vi "VIPM_Get Spec File Paths.vi"() -> (2 "Success?":bool, 3 "Spec Paths":path[](array[path]))   [LabVIEW 2019, in "Project.Dependencies Finder.lvlib" / "Dependency Source_VIPM.lvclass"]
doc: "Returns the paths to all Spec files in the JKI\\VIPM\\Cache folder."
uses:
  Dependency Source_VIPM.lvclass
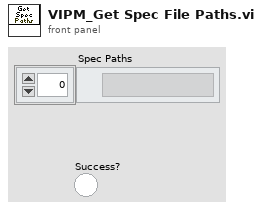
[diagram p1: front panel]
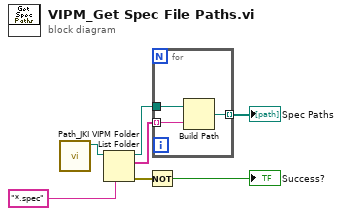
[diagram p0: block diagram]
diagram:
  n1 = call "Path_JKI VIPM Folder.vi"() -> ("JKI\\VIPM path"=w1:path)  [unwired: 10 in, 1 out]
  n2 = List Folder(path=w1, pattern="*.spec") -> (path out=w6:path, filenames=w5:string[], error out=w3:errorcluster)  [unwired: 2 in, 1 out]
  n3 = Not(x=w3) -> (.not. x?=→"Success?":bool)
  n4 = for {
    tunnel: w6 -> [w10]
    tunnel: w5 -> [w9] mode=indexing
    tunnel: [w8] -> w4 mode=indexing
    n5 = Build Path(base path=w10, name or relative path=w9) -> (appended path=w8:path)
  }
  "Spec Paths" <- w4
